vi "Average Readings Float.vi"(9 "Input Array Data U16":dbl[](array[numeric]), 11 "# of Points":u16) -> (3 "Average":dbl)   [LabVIEW 2010]
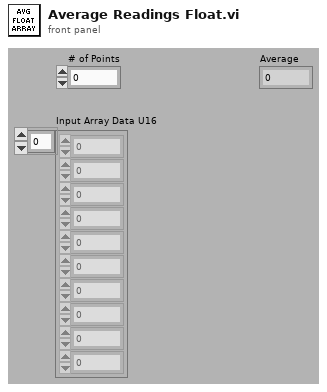
[diagram p1: front panel]
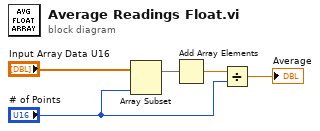
[diagram p0: block diagram]
diagram:
  n1 = Array Subset(array="Input Array Data U16", length="# of Points") -> (w4:dbl[])  [unwired: 1 in]
  n2 = Add Array Elements(numeric array=w4) -> (sum=w3:dbl)
  n3 = Divide(x=w3, y="# of Points") -> (x/y=→"Average":dbl)
